vi "Scope User Interface.vi"() -> ()   [LabVIEW 2023, in "GUI.lvlib" / "Diagnostic.lvlib"]
uses:
  Diagnostic.lvlib
  <instrlib>/niScope/Controls/niScope scalar measurement.ctl
  <instrlib>/niScope/Controls/niScope array measurement.ctl
panel:
  in  "String":string
  in  "Stop":bool caption="Blank"
  in  "Apply":bool caption="Blank"
  in  "Scope Operation":T1(tab)
  in  "Scope":refnum<k15>="PXI1Slot2"
  in  "Trigger Modifier":i32(ring)=1 caption="Measurement Function (DC Volts)" items=["None"=1, "Auto Trigger"=2]
  in  "Referance Position":dbl=1e-06 caption="Absolute Resolution (1E-6)" format="%.2p"
  in  "Trigger Delay (s)":dbl=1e-06 caption="Absolute Resolution (1E-6)" format="%.2p"
  in  "Enforce Realtime":bool=TRUE
  in  "Record Length":dbl=1e-06 caption="Absolute Resolution (1E-6)" format="%.2p"
  in  "Sample Rate":dbl=1e-06 caption="Absolute Resolution (1E-6)" format="%.2p"
  in  "Acquire":i32(ring)=1 caption="Measurement Function (DC Volts)" items=["AC", "DC", "Ground"]
  in  "Bandwidth (Hz)":dbl=1e-06 caption="Absolute Resolution (1E-6)" format="%.2p"
  in  "Probe atten":dbl=1e-06 caption="Absolute Resolution (1E-6)" format="%.2p"
  in  "Channel Name":string(combo)="0"
  in  "Offset (V)":dbl=1e-06 caption="Absolute Resolution (1E-6)" format="%.2p"
  in  "Range (V)":dbl
  in  "Coupling":i32(ring)=1 caption="Measurement Function (DC Volts)" items=["AC", "DC", "Ground"]
  in  "Input Impedance":u32(ring)=1 caption="Measurement Function (DC Volts)" items=["1 Mega Ohm", "75 Ohm", "50 Ohm"]
  in  "Trigger Type":T2(tab)
  in  "Trigger Source (Edge)":string(combo)="0" caption="Trigger Source"
  in  "Trigger Level (Edge)":dbl
  in  "Trigger Slope (Edge)":u16(ring)=1 caption="Measurement Function (DC Volts)" items=["Positive", "Negative"]
  in  "Trigger Coupling (Edge)":u32(ring)=1 caption="Measurement Function (DC Volts)" items=["AC"=0, "DC"=1, "HF Reject"=3, "LF Reject"=4, "AC Plus HF Reject"=1001]
  in  "Trigger Slope (Dig)":u16(ring)=1 caption="Measurement Function (DC Volts)" items=["Positive", "Negative"]
  in  "Trigger Source (Dig)":string(combo)="0" caption="Trigger Source"
  in  "Trigger Coupling (Win)":u32(ring)=1 caption="Measurement Function (DC Volts)" items=["AC"=0, "DC"=1, "HF Reject"=3, "LF Reject"=4, "AC Plus HF Reject"=1001]
  in  "Window High Level":dbl=1e-06 caption="Absolute Resolution (1E-6)" format="%.2p"
  in  "Window Low Level":dbl=1e-06 caption="Absolute Resolution (1E-6)" format="%.2p"
  in  "Window Mode":i32(ring)=1 caption="Measurement Function (DC Volts)" items=["Entering", "Leaving"]
  in  "Trigger Source (Win)":string(combo)="0" caption="Trigger Source"
  in  "Hysteresis":dbl
  in  "Trigger Source (Hys)":string(combo)="0" caption="Trigger Source"
  in  "Trigger Level (Hys)":dbl
  in  "Trigger Coupling (Hys)":u32(ring)=1 caption="Measurement Function (DC Volts)" items=["AC"=0, "DC"=1, "HF Reject"=3, "LF Reject"=4, "AC Plus HF Reject"=1001]
  in  "Trigger Slope (Hys)":u16(ring)=1 caption="Measurement Function (DC Volts)" items=["Positive", "Negative"]
  out "Measurement":dbl
  out "Waveform Graph - Light":waveform(dbl)(graph)
  in  "Measure":T3(tab)
  in  "scalar measurement":T4=4000 caption="Scalar Measurement" items=["None"=4000, "Frequency"=2, "Average Frequency"=1016, "FFT Frequency"=1008, "Period"=3, "Average Period"=1015, "Rise Time"=0, "Fall Time"=1, "Rising Slew Rate"=1010, "Falling Slew Rate"=1011, "Overshoot"=18, "Preshoot"=19, "Voltage RMS"=4, "Voltage Cycle RMS"=16, "AC Estimate"=1012, "FFT Amplitude"=1009, "Voltage Average"=10, "Voltage Cycle Average"=17, "DC Estimate"=1013, "Voltage Max"=6, "Voltage Min"=7, "Voltage Peak-to-Peak"=5, "Voltage High"=8, "Voltage Low"=9, "Voltage Amplitude"=15, "Voltage Top"=1007, "Voltage Base"=1006, "Voltage Base-to-Top"=1017, "Negative Width"=11, "Positive Width"=12, "Negative Duty Cycle"=13, "Positive Duty Cycle"=14, "Integral"=1005, "Area"=1003, "Cycle Area"=1004, "Time Delay"=1014, "Phase Delay"=1018, "Low Ref Volts"=1000, "Mid Ref Volts"=1001, "High Ref Volts"=1002, "Volt. Hist. Mean"=2000, "Volt. Hist. Stdev"=2001, "Volt. Hist. Median"=2003, "Volt. Hist. Mode"=2010, "Volt. Hist. Max"=2005, "Volt. Hist. Min"=2006, "Volt. Hist. Peak-to-Peak"=2002, "Volt. Hist. Mean + Stdev"=2007, "Volt. Hist. Mean + 2 Stdev"=2008, "Volt. Hist. Mean + 3 Stdev"=2009, "Volt. Hist. Hits"=2004, "Volt. Hist. New Hits"=2011, "Time Hist. Mean"=3000, "Time Hist. Stdev"=3001, "Time Hist. Median"=3003, "Time Hist. Mode"=3010, "Time Hist. Max"=3005, "Time Hist. Min"=3006, "Time Hist. Peak-to-Peak"=3002, "Time Hist. Mean + Stdev"=3007, "Time Hist. Mean + 2 Stdev"=3008, "Time Hist. Mean + 3 Stdev"=3009, "Time Hist. Hits"=3004, "Time Hist. New Hits"=3011]
  in  "Array Measurement":T5=4000 items=["None"=4000, "Last Acq. Histogram"=4001, "Multi Acq. Voltage Histogram"=4004, "Multi Acq. Time Histogram"=4005, "Multi Acq. Average"=4016, "Polynomial Interpolation"=4011, "Array Integral"=4006, "Derivative"=4007, "Inverse"=4008, "Multiply Channels"=4012, "Add Channels"=4013, "Subtract Channels"=4014, "Divide Channels"=4015, "Array Offset"=4025, "Array Gain"=4026, "Hanning Window"=4009, "Flat Top Window"=4010, "Hamming Window"=4020, "Triangle Window"=4023, "Blackman Window"=4024, "FIR Windowed Filter"=4021, "Bessel IIR Filter"=4022, "Butterworth IIR Filter"=4017, "Chebyshev IIR Filter"=4018, "FFT Phase Spectrum"=4002, "FFT Amp. Spectrum (Volts RMS)"=4003, "FFT Amp. Spectrum (dB)"=4019]
  # "Digital Oscilloscope"
  # "Operation:"
  # "Self Test is Enabled by selecting this opeartion"
  # "Vertical"
  # "Trigger Mode"
  # "Horizontal"
  # "General Trigger Settings"
  # "Scope Close Operation will be executing \nby selecting this opeartion"
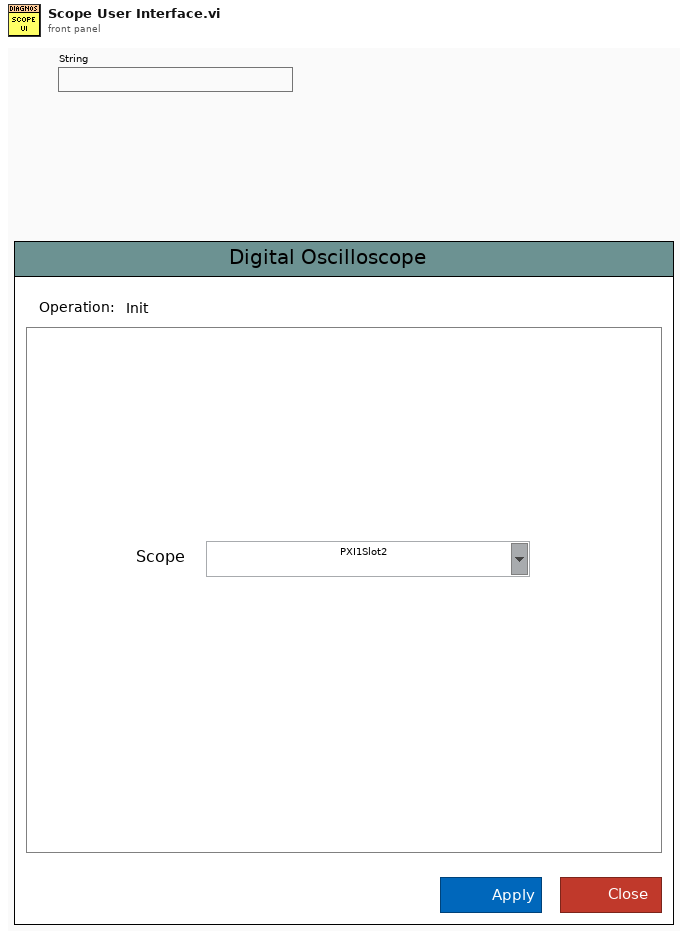
[diagram p1: front panel]
types:
  T1 = enum32{"Init", "Self Test", "Configure", "Measure", "Generate", "Close"}
  T2 = enum32{"Immediate", "Edge", "Digital", "Window", "Hysteresis"}
  T3 = enum32{"Scalar Measurement", "Array Measurement"}
  T4 = typedef "niScope scalar measurement.ctl" = i32
  T5 = typedef "niScope array measurement.ctl" = i32
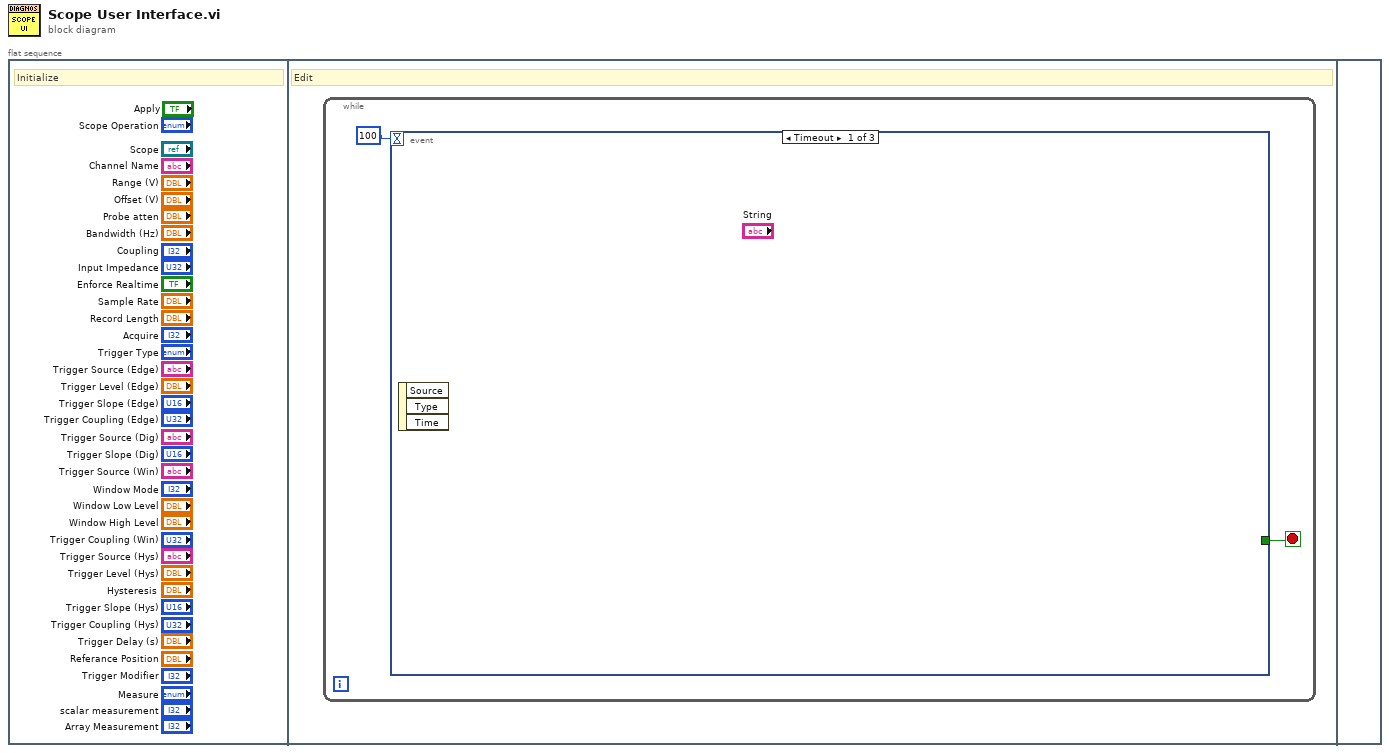
[diagram p0: block diagram]
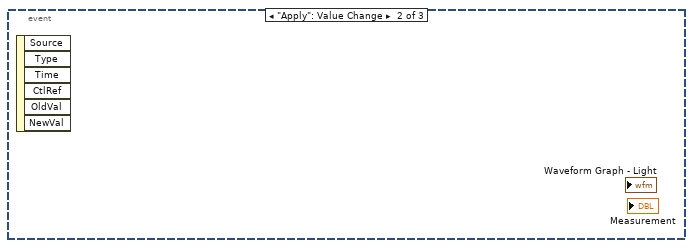
[diagram p2: hidden frame]
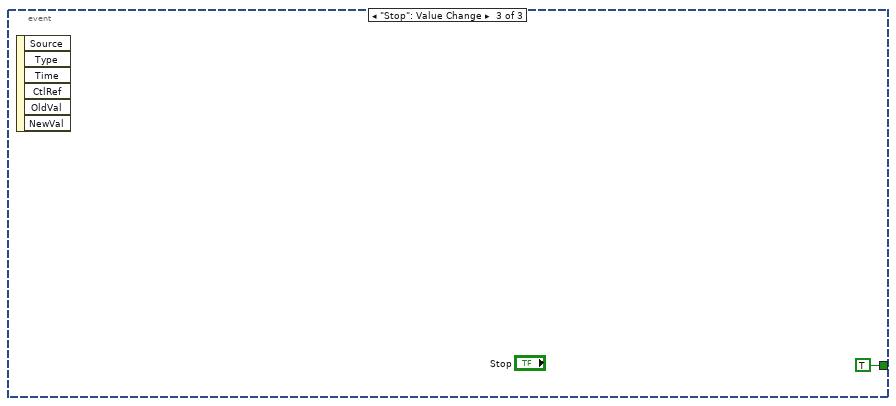
[diagram p3: hidden frame]
diagram:
  n1 = flat-sequence {
    frame #0 {
      # "Initialize"
    }
    frame #1 {
      # "Edit"
      n2 = while {
        stop <- w1 stop-if-true
        n3 = event shown="[0] Timeout" {
          selector: _ -> [_ _ _]
          dyn-events: _ -> [_ _ _]
          timeout: 100 -> [_ _ _]
          tunnel: [_ _ TRUE ("Stop")] -> w1
          event Timeout {
            n4 = event-data() -> ()  [unwired: 1 in, 3 out]
          }
          event "Apply": Value Change {
            n5 = event-data() -> ()  [unwired: 1 in, 6 out]
          }
          event "Stop": Value Change {
            n6 = event-data() -> ()  [unwired: 1 in, 6 out]
          }
        }
      }
    }
    frame #2 {
    }
  }
